vi "Set Channel Mode.vi"(8 "error in (no error)":errorcluster, 9 "Channel List(\"\")":string, 10 "Channel Mode (0: Input)":i32(ring) items=["Input", "Output", "Rising", "Falling", "Rising_reset", "Falling_reset"], 11 "VISA resource name":refnum<visa-resource-name>) -> (0 "error out":errorcluster, 3 "VISA resource name out":refnum<visa-resource-name>)   [LabVIEW 2016, in "Keithley DMM6500 DAQ6500 Series.lvlib"]
doc: "Sets the mode of operation of a channel."
uses:
  Keithley DMM6500 DAQ6500 Series.lvlib
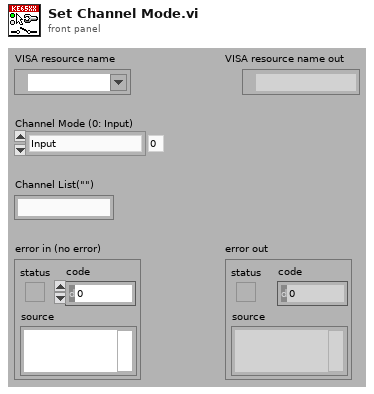
[diagram p1: front panel]
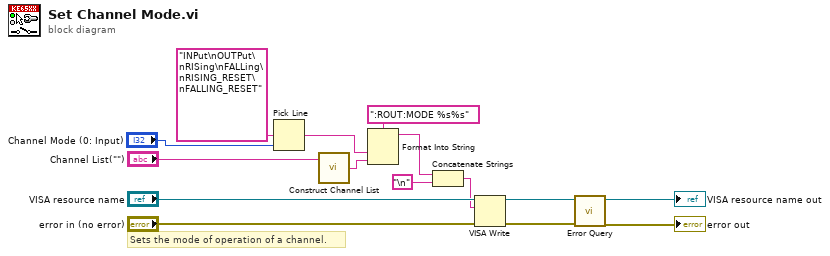
[diagram p0: block diagram]
diagram:
  # "Sets the mode of operation of a channel."
  n1 = Pick Line(multi-line string="INPut\nOUTPut\nRISing\nFALLing\nRISING_RESET\nFALLING_RESET", line index="Channel Mode (0: Input)") -> (output string=w3:string)  [unwired: 1 in]
  n2 = call "Construct Channel List.vi"("Channel List"="Channel List(\"\")") -> ("Channel List String"=w5:string)  [unwired: 2 in]
  n3 = Format Into String(format string=":ROUT:MODE %s%s", w3, w5) -> (resulting string=w7:string)  [unwired: 2 in, 1 out]
  n4 = Concatenate Strings(w7, "\n") -> (w8:string)
  n5 = VISA Write(VISA resource name="VISA resource name", write buffer=w8, error in (no error)="error in (no error)") -> (VISA resource name out=w12:refnum<visa-resource-name>, error out=w11:errorcluster)  [unwired: 1 out]
  n6 = call "Error Query.vi"("error in (no error)"=w11, "VISA resource name"=w12) -> ("error out"=→"error out":errorcluster, "VISA resource name out"=→"VISA resource name out":refnum<visa-resource-name>)  [unwired: 6 in, 2 out]
